vi "AutoHandler.vi"(8 "error in (no error)":errorcluster) -> (0 "Severity":string, 1 "Stop":bool, 2 "Abort":bool, 3 "Continue":bool)   [LabVIEW 2018]
panel:
  # "The General handler currently looks for the following severities:\n\n     Fatal  \n     Critical\n     Abort (when a process or state machine needs to stop but   the application can continue.\n     Warning\n     Inform\n     Log (no dialog will be launched)"
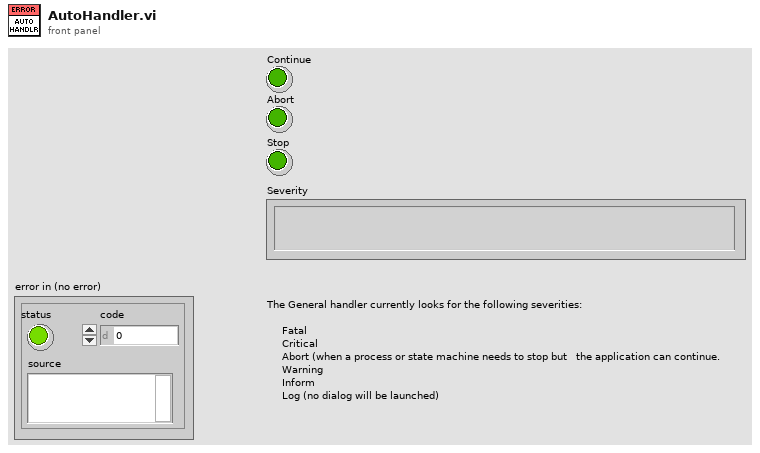
[diagram p1: front panel]
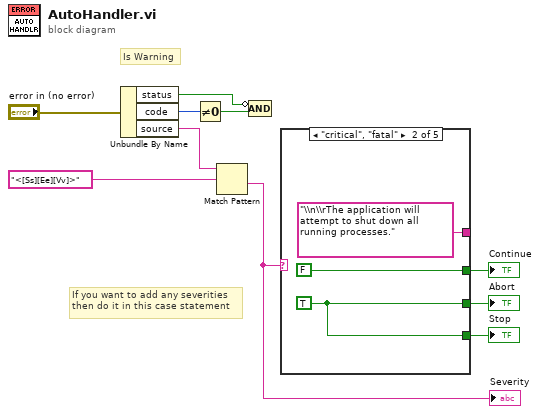
[diagram p0: block diagram]
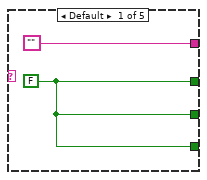
[diagram p2: hidden frame]
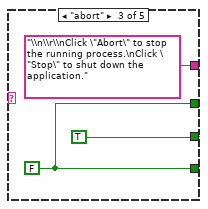
[diagram p3: hidden frame]
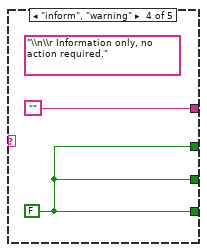
[diagram p4: hidden frame]
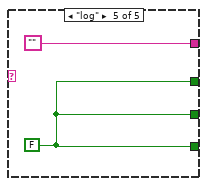
[diagram p5: hidden frame]
diagram:
  # "If you want to add any severities\nthen do it in this case statement"
  # "Is Warning"
  n1 = Unbundle By Name("error in (no error)") -> ("status"=w8:bool, "code"=w5:i32, "source"=w6:string)
  n2 = Not Equal To 0?(x=w5) -> (x != 0?=w9:bool)
  n3 = Match Pattern(string=w6, regular expression="<[Ss][Ee][Vv]>") -> (after substring=w4:string)  [unwired: 1 in, 3 out]
  "Severity" <- w4
  n4 = Compound Arithmetic op=AND(invert w8, w9) -> ()  [unwired: 1 out]
  n5 = case shown="\"critical\", \"fatal\"" w4 {
    tunnel: ["" "\\n\\rThe application will attempt to shut down all running processes." "\\n\\r\\nClick \"Abort\" to stop the running process.\nClick \"Stop\" to shut down the application." "" ""] -> _
    tunnel: [w11 FALSE ("Continue") w16 w19 w21] -> w3
    tunnel: [w11 w14 TRUE ("Continue") w19 w21] -> w2
    tunnel: [w11 w14 w16 w19 w21] -> w1
    frame Default {
      w11 = FALSE ("Continue")
    }
    frame "critical", "fatal" {
      w14 = TRUE ("Continue")
    }
    frame "abort" {
      w16 = FALSE ("Continue")
    }
    frame "inform", "warning" {
      (unwired) "\\n\\r Information only, no action required."
      w19 = FALSE ("Continue")
    }
    frame "log" {
      w21 = FALSE ("Continue")
    }
  }
  "Abort" <- w2
  "Continue" <- w3
  "Stop" <- w1
